vi "Pod Health Status.vi"(10 "Telemetry":T1 {"Brake Pressure (PSI)" scale=0.0..1000.0; "Maglock 4 (mm)" scale=0.0..15.0; "Maglock 3 (mm)" scale=0.0..15.0; "Maglock 2 (mm)" scale=0.0..15.0; "Maglock 1 (mm)" scale=0.0..15.0; "ToF 4 (mm)" scale=0.0..100.0; "ToF 3 (mm)" scale=0.0..100.0; "ToF 2 (mm)" scale=0.0..100.0; "ToF 1 (mm)" scale=0.0..100.0; "Low Pressure (PSI)" scale=0.0..1000.0; "Med. Pressure (PSI)" scale=0.0..1000.0; "High Pressure (PSI)" scale=0.0..1000.0; "Backup Batt. (V)" scale=0.0..15.0; "Prim. Batt. (V)" scale=0.0..15.0; "Mag Brake (mA)" scale=0.0..500.0; "Friction Brake (mA)" scale=0.0..500.0}, 11 "Pod Health Configuration":T2={"Power"={"Brake Max (mA)"=400.0, "Brake Min (mA)"=200.0, "Batt. Min (V)"=11.5, "Batt. Max (V)"=13.0}, "Pressure"={"HP Max (PSI)"=3000.0, "HP Min (PSI)"=2000.0, "MP Max (PSI)"=350.0, "MP Min (PSI)"=250.0, "LP Max (PSI)"=55.0, "LP Min (PSI)"=45.0, "BP Max (PSI)"=250.0, "BP Min (PSI)"=150.0}, "Position"={"Maglock Max (mm)"=3.0, "Maglock Min (mm)"=0.0, "Lev. Min (mm)"=8.0, "Lev. Max (mm)"=15.0}}) -> (2 "Pod Health":T3)   [LabVIEW 2014]
uses:
  Type Defs/PodHealth.ctl
  Type Defs/PodHealthConfig.ctl
  Type Defs/Telemetry.ctl
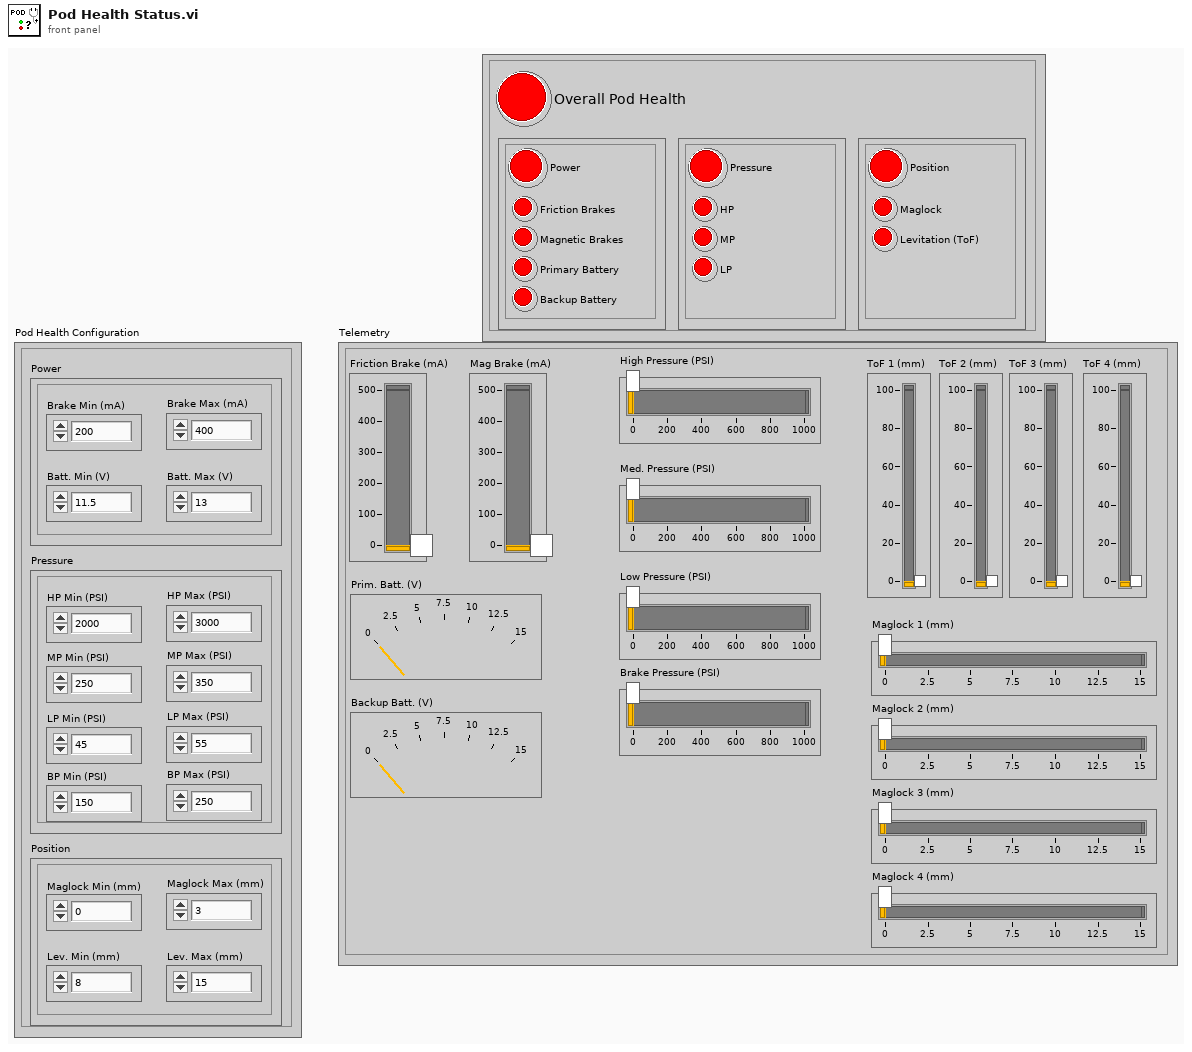
[diagram p1: front panel]
types:
  T1 = typedef "Telemetry.ctl" = cluster{"Friction Brake (mA)":dbl, "Mag Brake (mA)":dbl, "Prim. Batt. (V)":dbl, "Backup Batt. (V)":dbl, "High Pressure (PSI)":dbl, "Med. Pressure (PSI)":dbl, "Low Pressure (PSI)":dbl, "Brake Pressure (PSI)":dbl, "ToF 1 (mm)":dbl, "ToF 2 (mm)":dbl, "ToF 3 (mm)":dbl, "ToF 4 (mm)":dbl, "Maglock 1 (mm)":dbl, "Maglock 2 (mm)":dbl, "Maglock 3 (mm)":dbl, "Maglock 4 (mm)":dbl}
  T2 = typedef "PodHealthConfig.ctl" = cluster{"Power":cluster{"Brake Max (mA)":dbl, "Brake Min (mA)":dbl, "Batt. Min (V)":dbl, "Batt. Max (V)":dbl}, "Pressure":cluster{"HP Max (PSI)":dbl, "HP Min (PSI)":dbl, "MP Max (PSI)":dbl, "MP Min (PSI)":dbl, "LP Max (PSI)":dbl, "LP Min (PSI)":dbl, "BP Max (PSI)":dbl, "BP Min (PSI)":dbl}, "Position":cluster{"Maglock Max (mm)":dbl, "Maglock Min (mm)":dbl, "Lev. Min (mm)":dbl, "Lev. Max (mm)":dbl}}
  T3 = typedef "PodHealth.ctl" = cluster{"Overall Pod Health":bool, "Power":cluster{"Power":bool, "Friction Brakes":bool, "Magnetic Brakes":bool, "Primary Battery":bool, "Backup Battery":bool}, "Pressure":cluster{"Pressure":bool, "HP":bool, "MP ":bool, "LP":bool}, "Position":cluster{"Position":bool, "Maglock":bool, "Levitation (ToF)":bool}}
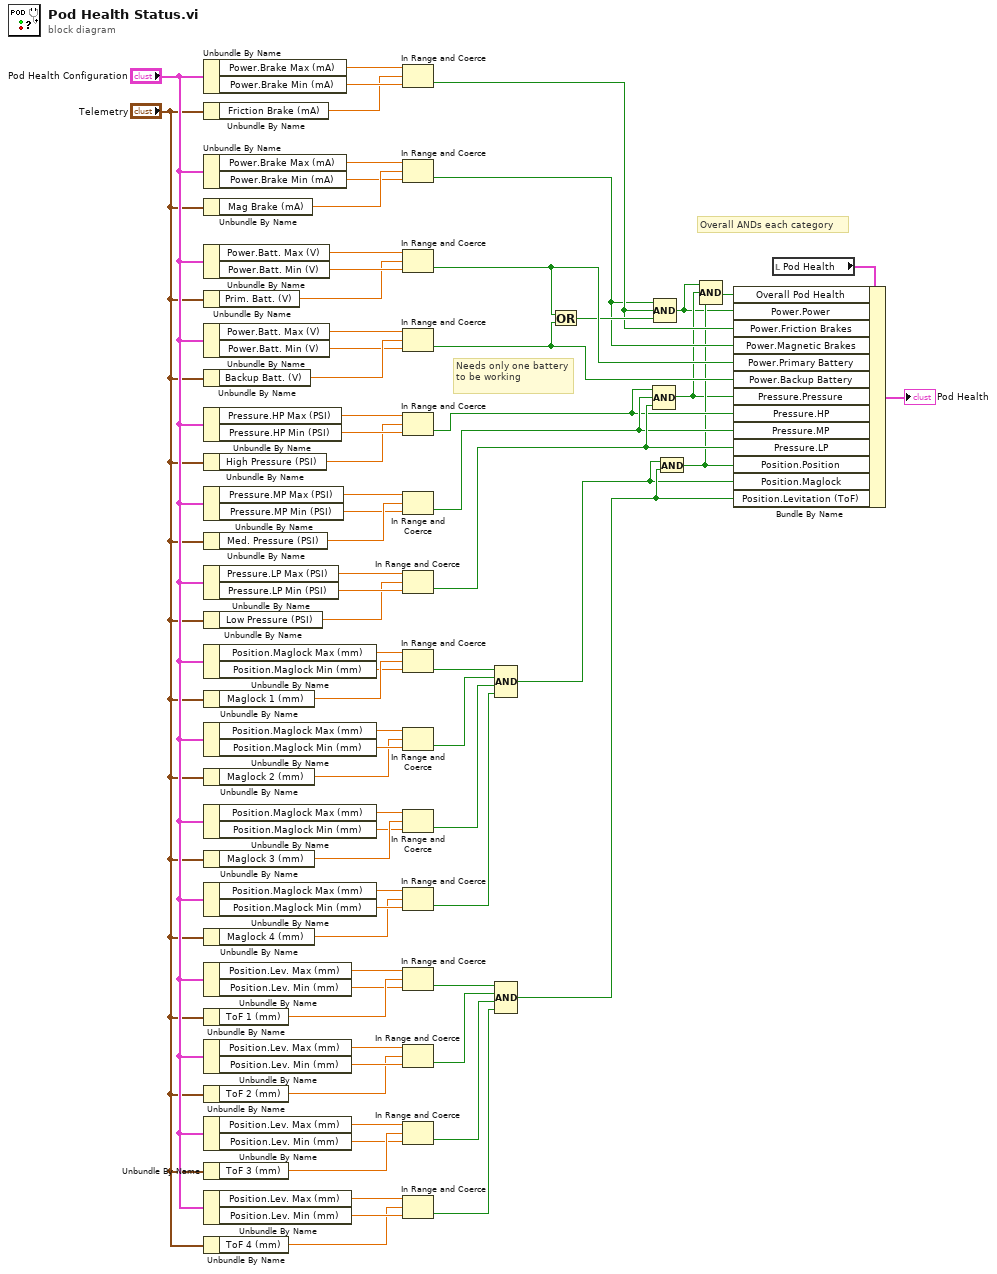
[diagram p0: block diagram]
diagram:
  # "Overall ANDs each category"
  # "Needs only one battery to be working"
  n1 = Unbundle By Name("Pod Health Configuration") -> ("Power.Brake Max (mA)"=w71:dbl, "Power.Brake Min (mA)"=w70:dbl)
  n2 = Unbundle By Name("Telemetry") -> ("Friction Brake (mA)"=w69:dbl)
  n3 = Unbundle By Name("Pod Health Configuration") -> ("Power.Brake Max (mA)"=w66:dbl, "Power.Brake Min (mA)"=w67:dbl)
  n4 = Unbundle By Name("Telemetry") -> ("Mag Brake (mA)"=w68:dbl)
  n5 = Unbundle By Name("Pod Health Configuration") -> ("Power.Batt. Max (V)"=w63:dbl, "Power.Batt. Min (V)"=w62:dbl)
  n6 = Unbundle By Name("Telemetry") -> ("Prim. Batt. (V)"=w61:dbl)
  n7 = Unbundle By Name("Pod Health Configuration") -> ("Power.Batt. Max (V)"=w58:dbl, "Power.Batt. Min (V)"=w59:dbl)
  n8 = Unbundle By Name("Telemetry") -> ("Backup Batt. (V)"=w60:dbl)
  n9 = Unbundle By Name("Pod Health Configuration") -> ("Pressure.HP Max (PSI)"=w57:dbl, "Pressure.HP Min (PSI)"=w56:dbl)
  n10 = Unbundle By Name("Telemetry") -> ("High Pressure (PSI)"=w55:dbl)
  n11 = Unbundle By Name("Pod Health Configuration") -> ("Pressure.MP Max (PSI)"=w52:dbl, "Pressure.MP Min (PSI)"=w53:dbl)
  n12 = Unbundle By Name("Telemetry") -> ("Med. Pressure (PSI)"=w54:dbl)
  n13 = Unbundle By Name("Pod Health Configuration") -> ("Pressure.LP Max (PSI)"=w51:dbl, "Pressure.LP Min (PSI)"=w50:dbl)
  n14 = Unbundle By Name("Telemetry") -> ("Low Pressure (PSI)"=w49:dbl)
  n15 = Unbundle By Name("Pod Health Configuration") -> ("Position.Maglock Max (mm)"=w46:dbl, "Position.Maglock Min (mm)"=w47:dbl)
  n16 = Unbundle By Name("Telemetry") -> ("Maglock 1 (mm)"=w48:dbl)
  n17 = Unbundle By Name("Pod Health Configuration") -> ("Position.Maglock Max (mm)"=w45:dbl, "Position.Maglock Min (mm)"=w44:dbl)
  n18 = Unbundle By Name("Telemetry") -> ("Maglock 2 (mm)"=w43:dbl)
  n19 = Unbundle By Name("Pod Health Configuration") -> ("Position.Maglock Max (mm)"=w40:dbl, "Position.Maglock Min (mm)"=w41:dbl)
  n20 = Unbundle By Name("Telemetry") -> ("Maglock 3 (mm)"=w42:dbl)
  n21 = Unbundle By Name("Pod Health Configuration") -> ("Position.Maglock Max (mm)"=w39:dbl, "Position.Maglock Min (mm)"=w38:dbl)
  n22 = Unbundle By Name("Telemetry") -> ("Maglock 4 (mm)"=w37:dbl)
  n23 = Unbundle By Name("Pod Health Configuration") -> ("Position.Lev. Max (mm)"=w34:dbl, "Position.Lev. Min (mm)"=w35:dbl)
  n24 = Unbundle By Name("Telemetry") -> ("ToF 1 (mm)"=w36:dbl)
  n25 = Unbundle By Name("Pod Health Configuration") -> ("Position.Lev. Max (mm)"=w33:dbl, "Position.Lev. Min (mm)"=w32:dbl)
  n26 = Unbundle By Name("Telemetry") -> ("ToF 2 (mm)"=w31:dbl)
  n27 = Unbundle By Name("Pod Health Configuration") -> ("Position.Lev. Max (mm)"=w28:dbl, "Position.Lev. Min (mm)"=w29:dbl)
  n28 = Unbundle By Name("Telemetry") -> ("ToF 3 (mm)"=w30:dbl)
  n29 = Unbundle By Name("Pod Health Configuration") -> ("Position.Lev. Max (mm)"=w27:dbl, "Position.Lev. Min (mm)"=w26:dbl)
  n30 = Unbundle By Name("Telemetry") -> ("ToF 4 (mm)"=w25:dbl)
  n31 = In Range and Coerce(upper limit=w71, x=w69, lower limit=w70) -> (In Range?=w6:bool)  [unwired: 1 out]
  n32 = In Range and Coerce(upper limit=w66, x=w68, lower limit=w67) -> (In Range?=w5:bool)  [unwired: 1 out]
  n33 = In Range and Coerce(upper limit=w63, x=w61, lower limit=w62) -> (In Range?=w8:bool)  [unwired: 1 out]
  n34 = In Range and Coerce(upper limit=w58, x=w60, lower limit=w59) -> (In Range?=w9:bool)  [unwired: 1 out]
  n35 = In Range and Coerce(upper limit=w57, x=w55, lower limit=w56) -> (In Range?=w10:bool)  [unwired: 1 out]
  n36 = In Range and Coerce(upper limit=w52, x=w54, lower limit=w53) -> (In Range?=w11:bool)  [unwired: 1 out]
  n37 = In Range and Coerce(upper limit=w51, x=w49, lower limit=w50) -> (In Range?=w12:bool)  [unwired: 1 out]
  n38 = In Range and Coerce(upper limit=w46, x=w48, lower limit=w47) -> (In Range?=w22:bool)  [unwired: 1 out]
  n39 = In Range and Coerce(upper limit=w45, x=w43, lower limit=w44) -> (In Range?=w19:bool)  [unwired: 1 out]
  n40 = In Range and Coerce(upper limit=w40, x=w42, lower limit=w41) -> (In Range?=w20:bool)  [unwired: 1 out]
  n41 = In Range and Coerce(upper limit=w39, x=w37, lower limit=w38) -> (In Range?=w21:bool)  [unwired: 1 out]
  n42 = In Range and Coerce(upper limit=w34, x=w36, lower limit=w35) -> (In Range?=w18:bool)  [unwired: 1 out]
  n43 = In Range and Coerce(upper limit=w33, x=w31, lower limit=w32) -> (In Range?=w15:bool)  [unwired: 1 out]
  n44 = In Range and Coerce(upper limit=w28, x=w30, lower limit=w29) -> (In Range?=w16:bool)  [unwired: 1 out]
  n45 = In Range and Coerce(upper limit=w27, x=w25, lower limit=w26) -> (In Range?=w17:bool)  [unwired: 1 out]
  n46 = Compound Arithmetic op=AND(w22, w19, w20, w21) -> (w13:bool)
  n47 = Compound Arithmetic op=AND(w18, w15, w16, w17) -> (w14:bool)
  n48 = Or(x=w8, y=w9) -> (x .or. y?=w7:bool)
  n49 = Compound Arithmetic op=AND(w10, w11, w12) -> (w2:bool)
  n50 = Compound Arithmetic op=AND(w5, w6, w7) -> (w1:bool)
  n51 = And(x=w13, y=w14) -> (x .and. y?=w3:bool)
  n52 = Compound Arithmetic op=AND(w1, w2, w3) -> (w4:bool)
  n53 = local read "Pod Health"() -> (w65:T3)
  n54 = Bundle By Name(cluster=w65, "Overall Pod Health"=w4, "Power.Power"=w1, "Power.Friction Brakes"=w6, "Power.Magnetic Brakes"=w5, "Power.Primary Battery"=w8, "Power.Backup Battery"=w9, "Pressure.Pressure"=w2, "Pressure.HP"=w10, "Pressure.MP"=w11, "Pressure.LP"=w12, "Position.Position"=w3, "Position.Maglock"=w13, "Position.Levitation (ToF)"=w14) -> (→"Pod Health":T3)
